vi "stringPosition.vi"(1 "Longitude":dbl format="%#.6g", 2 "Latitude":dbl format="%#.6g") -> (0 "StringPosition":string)   [LabVIEW 2015]
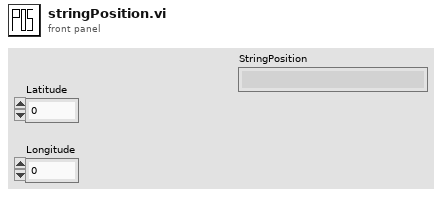
[diagram p1: front panel]
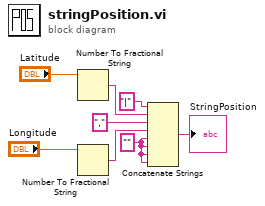
[diagram p0: block diagram]
diagram:
  w8 = ""
  n1 = Number To Fractional String(number="Latitude") -> (F-format string=w7:string)  [unwired: 3 in]
  n2 = Number To Fractional String(number="Longitude") -> (F-format string=w5:string)  [unwired: 3 in]
  n3 = Concatenate Strings("|", w7, ",", w5, w8, w8, w8, w8) -> (→"StringPosition":string)
